vi "FTW-Ether-Construct.vi"(5 "FTW Ether Configuration":string="{\n  \"ApplicationName\": \"Featherweight Application\",\n  \"ApplicationVersion\": \"0.1.0-1\",\n  \"LoggerAddress\": \"inproc://*\",\n  \"LoggerName\": \"Log\",\n  \"LoggerDirectory\": \"[UserAppData]\\\\Featherweight\\\\Logs\",\n  \"LoggerDiskThrashDelay\": 200\n}", 11 "error in":errorcluster) -> (15 "error out":errorcluster)   [LabVIEW 2015, in "FTW-Ether.lvclass"]
uses:
  FTW-Ether.lvclass
  FTW-Ether-Connections-Action.ctl
  FTW-Ether-Instance.vi
panel:
  # "Inputs"
  # "Outputs"
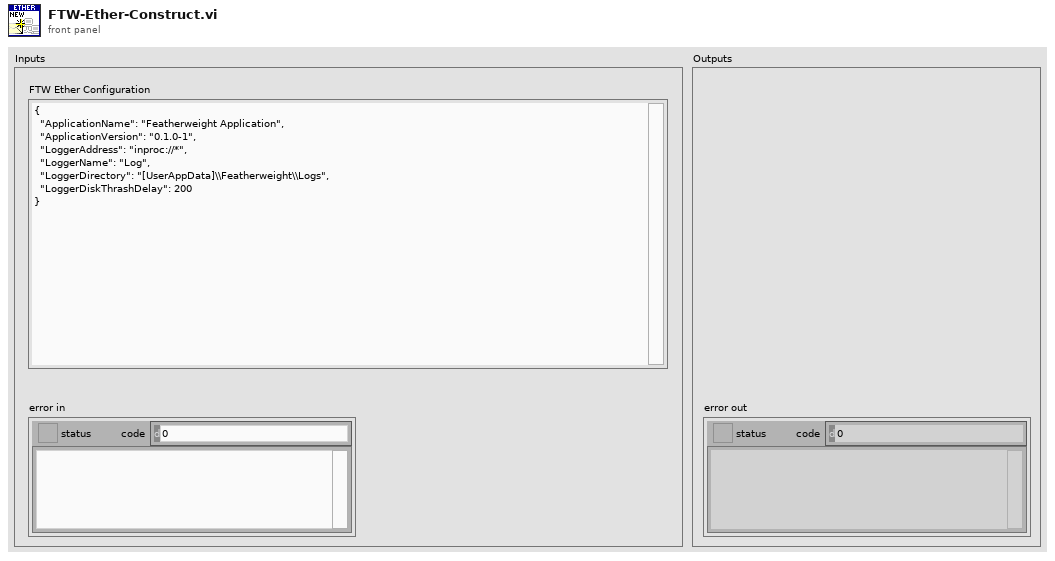
[diagram p1: front panel]
types:
  T1 = typedef "FTW-Ether.lvclass/FTW-Ether-Connections-Action.ctl" = enum8{"Query", "Add", "Reset"}
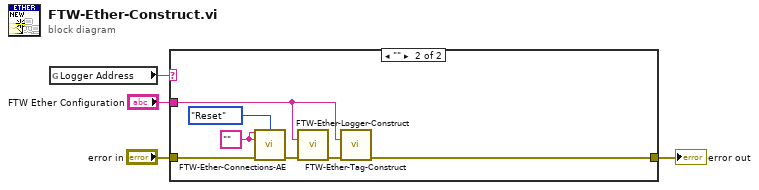
[diagram p0: block diagram]
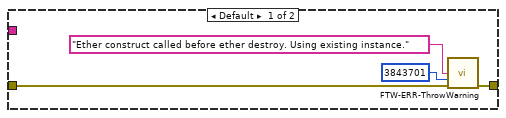
[diagram p2: hidden frame]
diagram:
  n1 = global read "FTW-Ether-Instance.vi" "Logger Address"() -> (w1:string)
  n2 = case shown="\"\"" w1 {
    tunnel: "FTW Ether Configuration" -> [_ w9]
    tunnel: "error in" -> [w8 w13]
    tunnel: [w7 w10] -> w2
    frame Default {
      n3 = call "FTW-ERR-ThrowWarning.vi"("Warning Message"="Ether construct called before ether destroy. Using existing instance.", "Error Code"=3843701, "error in"=w8) -> ("error out"=w7:errorcluster)  [unwired: 12 in]
    }
    frame "" {
      w14 = "" ("empty string")
      n4 = call "FTW-Ether-Connections-AE.vi"("Connection"=w14, "Action"=FTW-Ether-Connections-Action."Reset", "Address"=w14, "error in"=w13) -> ("error out"=w12:errorcluster)  [unwired: 10 in, 1 out]
      n5 = call "FTW-Ether-Logger-Construct.vi"("FTW Ether Configuration"=w9, "error in"=w12) -> ("error out"=w11:errorcluster)  [unwired: 13 in]
      n6 = call "FTW-Ether-Tag-Construct.vi"("FTW Ether Configuration"=w9, "error in"=w11) -> ("error out"=w10:errorcluster)  [unwired: 13 in]
    }
  }
  "error out" <- w2
